vi "solar_misc Parse CSV.vi"(0 "CSV String":string) -> (6 "2D Array":string[][](array[string]))   [LabVIEW 2018]
doc: "This parses a comma separated value table into a 2d array."
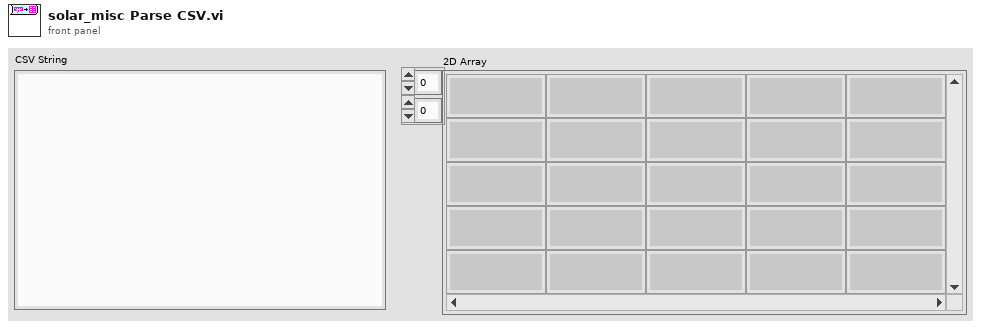
[diagram p1: front panel]
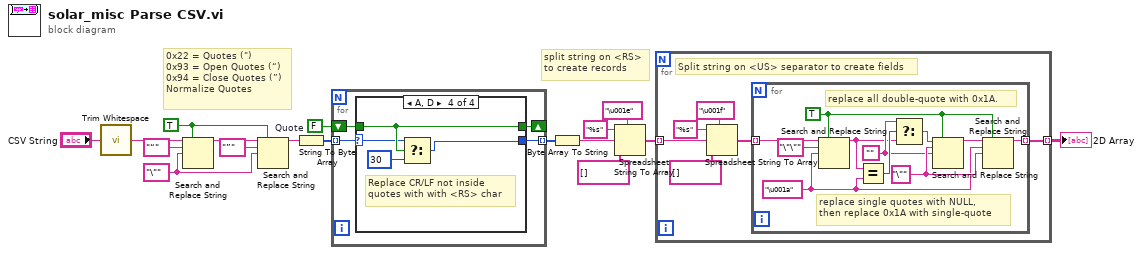
[diagram p0: block diagram]
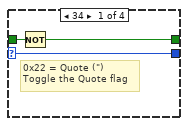
[diagram p2: hidden frame]
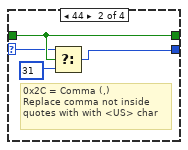
[diagram p3: hidden frame]
diagram:
  w12 = FALSE  # Quote
  w13 = TRUE ("replace all? (F)")
  w15 = "\"" ("replace string (\"\")")
  # "split string on <RS>\nto create records"
  # "0x22 = Quotes (\")\n0x93 = Open Quotes (“)\n0x94 = Close Quotes (”)\nNormalize Quotes"
  n1 = call <vilib>:"Trim Whitespace.vi"("string"="CSV String") -> ("trimmed string"=w1:string)  [unwired: 1 in]
  n2 = Search and Replace String(replace all?=w13, input string=w1, search string="“", replace string=w15) -> (result string=w16:string)  [unwired: 1 in, 6 out]
  n3 = Search and Replace String(replace all?=w13, input string=w16, search string="”", replace string=w15) -> (result string=w9:string)  [unwired: 1 in, 6 out]
  n4 = String To Byte Array(string=w9) -> (unsigned byte array=w11:u8[])
  n5 = for {
    tunnel: w11 -> [w18] mode=indexing
    shift-right: [w20] -> _
    shift-left: w12 -> [w21]
    tunnel: [w19] -> w10 mode=indexing
    n6 = case shown="A, D" w18 {
      selector: w18 -> [w23 w27 w29 w31]
      tunnel: w21 -> [w22 w28 w30 w34]
      tunnel: [w24 w28 w30 w34] -> w20
      tunnel: [w23 w25 w29 w32] -> w19
      frame 34 {
        # "0x22 = Quote (\")\nToggle the Quote flag"
        n7 = Not(x=w22) -> (.not. x?=w24:bool)
      }
      frame 44 {
        # "0x2C = Comma (,)\nReplace comma not inside \nquotes with with <US> char"
        n8 = Select(t=w27, s=w28, f=u8 31) -> (s? t:f=w25:u8)
      }
      frame Default {
      }
      frame 10, 13 {
        # "Replace CR/LF not inside \nquotes with with <RS> char"
        n9 = Select(t=w31, s=w34, f=u8 30) -> (s? t:f=w32:u8)
      }
    }
  }
  n10 = Byte Array To String(unsigned byte array=w10) -> (string=w4:string)
  n11 = Spreadsheet String To Array(delimiter (Tab)="\u001e", format string="%s", spreadsheet string=w4, array type (2D Dbl)=string[] []) -> (array=w7:string[])
  n12 = for {
    tunnel: w7 -> [w40] mode=indexing
    tunnel: [w37] -> w3 mode=indexing
    # "Split string on <US> separator to create fields"
    n13 = Spreadsheet String To Array(delimiter (Tab)="\u001f", format string="%s", spreadsheet string=w40, array type (2D Dbl)=string[] []) -> (array=w38:string[])
    n14 = for {
      tunnel: w38 -> [w41] mode=indexing
      tunnel: [w42] -> w37 mode=indexing
      w45 = ""
      w48 = "\"" ("input string")
      w49 = TRUE ("replace all? (F)")
      w47 = "\u001a" ("replace string (\"\")")
      # "replace single quotes with NULL,\nthen replace 0x1A with single-quote"
      # "replace all double-quote with 0x1A."
      n15 = Search and Replace String(replace all?=w49, input string=w41, search string="\"\"", replace string=w47) -> (result string=w44:string)  [unwired: 1 in, 6 out]
      n16 = Equal?(x=w44, y=w47) -> (x = y?=w46:bool)
      n17 = Select(t=w45, s=w46, f=w44) -> (s? t:f=w43:string)
      n18 = Search and Replace String(replace all?=w49, input string=w43, search string=w48, replace string=w45) -> (result string=w50:string)  [unwired: 1 in, 6 out]
      n19 = Search and Replace String(replace all?=w49, input string=w50, search string=w47, replace string=w48) -> (result string=w42:string)  [unwired: 2 in, 5 out]
    }
  }
  "2D Array" <- w3
